vi "Stop Core.vi"(10 "final error code":i32, 11 "Network Stream Reader in":refnum<class "Network Stream Reader.lvclass">) -> (3 "Network Stream Reader out":refnum<class "Network Stream Reader.lvclass">)   [LabVIEW 2014, in "Network Stream Reader.lvlib" / "Network Stream Reader.lvclass"]
doc: "(<B>Filename</B>: Actor Framework.lvlib:Actor.lvclass:Stop Core.vi)\n\nDefines what the actor does before it stops. Use the <B>final error code</B> input to determine whether the actor shut down in response to an error.\n\nBy default, this method does nothing. A descendant class may override it to define behavior, such as shutting down any processes the actor initiated in its override of the Actor Core method."
uses:
  Network Stream Reader.lvclass
  Network Stream Reader.lvclass/Network Stream Reader.ctl
  Network Stream/Network Stream/Network Stream.lvclass
panel:
  # "NStream Reader STOPED"
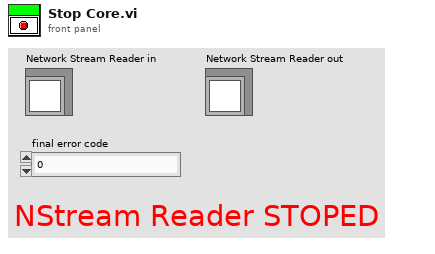
[diagram p1: front panel]
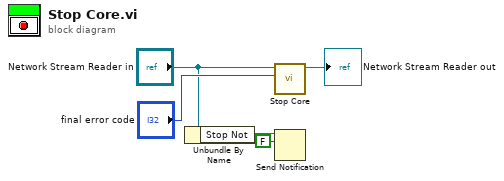
[diagram p0: block diagram]
diagram:
  n1 = Unbundle By Name("Network Stream Reader in") -> ("Stop Not"=w2:refnum<notifier>)
  n2 = call-parent "Stop Core.vi"("final error code"="final error code", "Network Stream in"="Network Stream Reader in") -> ("Network Stream out"=→"Network Stream Reader out":refnum<class "Network Stream Reader.lvclass">)  [unwired: 9 in]
  n3 = Send Notification(notification=FALSE, notifier=w2) -> ()  [unwired: 1 in, 2 out]
